vi "Bi Directional Trajectory.vi"(4 "Return Time":dbl, 6 "Go Time":dbl, 7 "Traj Start":bool, 10 "Trajectory Settings":T1) -> (1 "Return Next Time":dbl, 2 "Go Next Time":dbl, 3 "Output (mm)":dbl)   [LabVIEW 2021]
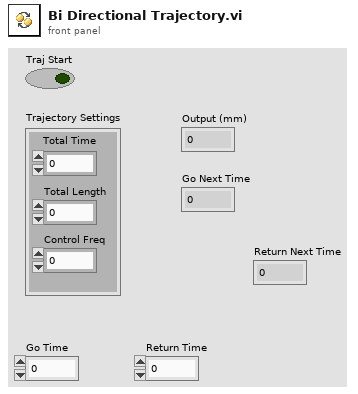
[diagram p1: front panel]
types:
  T1 = cluster{"Total Time":dbl, "Total Length":dbl, "Control Freq":dbl}
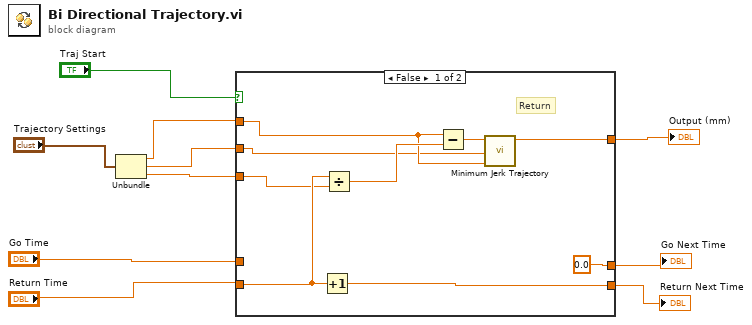
[diagram p0: block diagram]
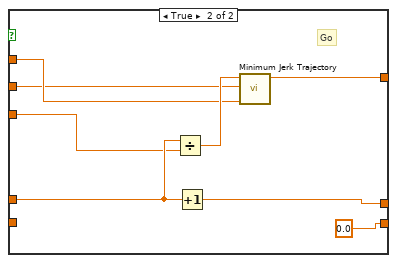
[diagram p2: hidden frame]
diagram:
  n1 = Unbundle("Trajectory Settings") -> ("Total Time"=w3:dbl, "Total Length"=w2:dbl, "Control Freq"=w1:dbl)
  n2 = case shown="False" "Traj Start" {
    tunnel: "Go Time" -> [_ w25]
    tunnel: [0.0 w27] -> w6
    tunnel: [w19 w24] -> w7
    tunnel: "Return Time" -> [w17 _]
    tunnel: [w11 0.0] -> w9
    tunnel: w3 -> [w14 w22]
    tunnel: w2 -> [w13 w21]
    tunnel: w1 -> [w12 w20]
    frame False {
      # "Return"
      n3 = Increment(x=w17) -> (x+1=w11:dbl)
      n4 = Divide(x=w17, y=w12) -> (x/y=w16:dbl)
      n5 = Subtract(x=w14, y=w16) -> (x-y=w15:dbl)
      n6 = call "Minimum Jerk Trajectory.vi"("total time"=w14, "total length"=w13, "t (sec)"=w15) -> ("ref_x (mm)"=w19:dbl)  [unwired: 7 in, 1 out]
    }
    frame True {
      # "Go"
      n7 = Divide(x=w25, y=w20) -> (x/y=w26:dbl)
      n8 = Increment(x=w25) -> (x+1=w27:dbl)
      n9 = call "Minimum Jerk Trajectory.vi"("total time"=w22, "total length"=w21, "t (sec)"=w26) -> ("ref_x (mm)"=w24:dbl)  [unwired: 7 in, 1 out]
    }
  }
  "Return Next Time" <- w9
  "Output (mm)" <- w7
  "Go Next Time" <- w6
